vi "Setup.vi"(8 "Error In":errorcluster, 11 "Address In":string) -> (0 "Error Out":errorcluster, 2 "Address Out":string, 3 "Sesssion":refnum<class "Session.lvclass">)   [LabVIEW 2018, in "Tests.lvlib" / "Known Hosts.lvlib"]
uses:
  Known Hosts.lvlib
  src/Toolkit/Session/Session.lvclass
  src/Toolkit/SSH/SSH.lvclass
  Tests.lvlib
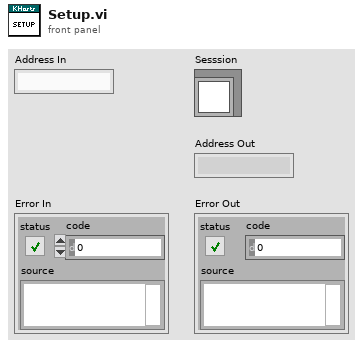
[diagram p1: front panel]
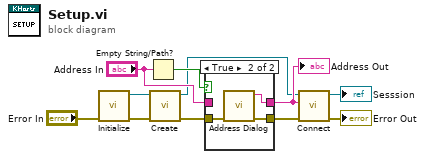
[diagram p0: block diagram]
diagram:
  n1 = call "Initialize.vi"("Error In"="Error In") -> ("Error Out"=w4:errorcluster, "SSH"=w1:refnum<class "SSH.lvclass">)  [unwired: 9 in]
  n2 = Empty String/Path?(string/path="Address In") -> (empty?=w7:bool)
  n3 = call "Create.vi"("Error In"=w4, "SSH"=w1) -> ("Error Out"=w9:errorcluster, "Sesssion"=w6:refnum<class "Session.lvclass">)  [unwired: 8 in]
  n4 = case shown="True" w7 {
    tunnel: w9 -> [w12 w16]
    tunnel: [w12 w15] -> w10
    tunnel: [w13 w14] -> w11
    tunnel: "Address In" -> [w13 _]
    frame False {
    }
    frame True {
      n5 = call "Address Dialog.vi"("Error In"=w16) -> ("Error Out"=w15:errorcluster, "Address Out"=w14:string)  [unwired: 9 in]
    }
  }
  "Address Out" <- w11
  n6 = call "Connect.vi"("Error In"=w10, "Address"=w11, "Session In"=w6) -> ("Error Out"=→"Error Out":errorcluster, "Sesssion Out"=→"Sesssion":refnum<class "Session.lvclass">)  [unwired: 7 in]
